vi "lightsource-emission-kill.vi"(1 "NKT Input":T1={"Emission"=FALSE, "Operation Mode"=FALSE, "Power Level"=5.0, "Feedback Level"=0.0, "Short Wavelength (nm)"=560, "Long Wavelength (nm)"=580, "UV Wavelength (nm)"=400} {"UV Wavelength (nm)" min=350 max=480 step=1; "Long Wavelength (nm)" min=400 max=850 step=1; "Short Wavelength (nm)" min=400 max=850 step=1; "Feedback Level" min=0.0 max=90.0 step=0.1 format="%.1f%%"; "Power Level" min=5.0 max=100.0 step=0.1 format="%.1f%%"}, 2 "VISA in":refnum<visa-resource-name>) -> (0 "lightsource init":bool=TRUE)   [LabVIEW 2015]
panel:
  in  "PortParameters":T2={"OpenPort"=FALSE, "ClosePort"=FALSE, "Baudrate"=115200, "Wait"=50, "ReadWrite"=TRUE}
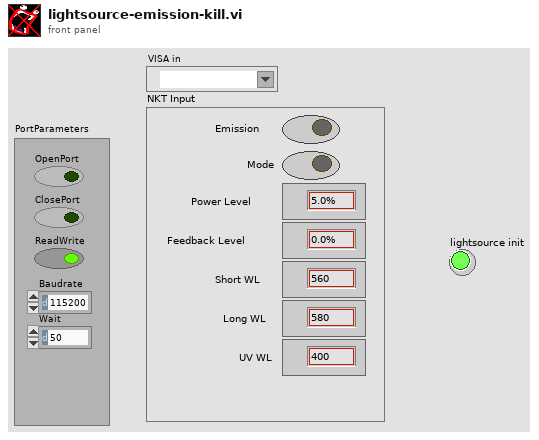
[diagram p1: front panel]
types:
  T1 = cluster{"Emission":bool, "Operation Mode":bool, "Power Level":dbl, "Feedback Level":dbl, "Short Wavelength (nm)":i32, "Long Wavelength (nm)":i32, "UV Wavelength (nm)":i32}
  T2 = cluster{"OpenPort":bool, "ClosePort":bool, "Baudrate":i32, "Wait":u16, "ReadWrite":bool}
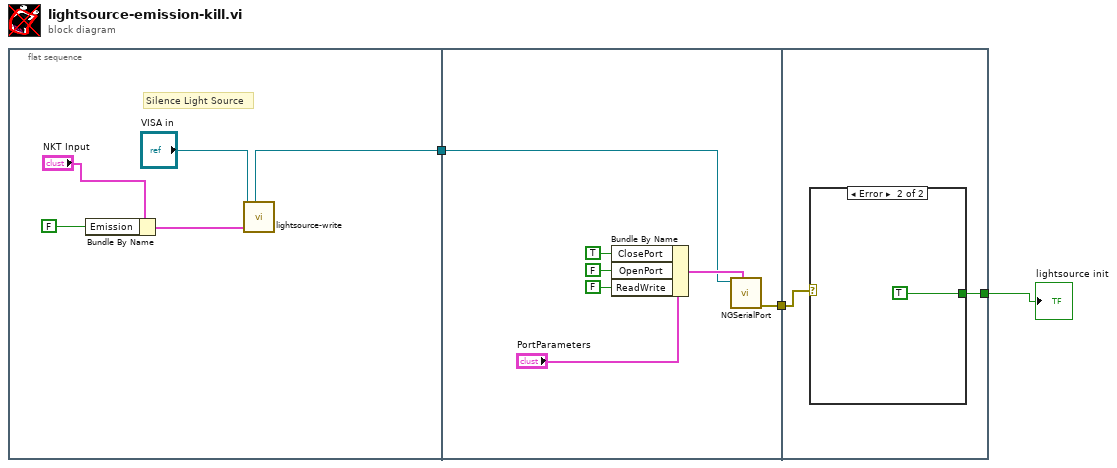
[diagram p0: block diagram]
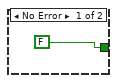
[diagram p2: hidden frame]
diagram:
  n1 = flat-sequence {
    tunnel: [w5] -> w3
    tunnel: w3 -> [w10]
    tunnel: [w9] -> w2
    tunnel: w2 -> [w17]
    tunnel: [w16] -> w1
    frame #0 {
      # "Silence Light Source"
      n2 = Bundle By Name(cluster="NKT Input", "Emission"=FALSE ("Emission On/Off")) -> (w7:T1)
      n3 = call "lightsource-write.vi"("VISA in"="VISA in", "NKT Input"=w7) -> ("VISA out"=w5:refnum<visa-resource-name>)  [unwired: 4 in, 2 out]
    }
    frame #1 {
      n4 = Bundle By Name(cluster="PortParameters", "ClosePort"=TRUE, "OpenPort"=FALSE, "ReadWrite"=FALSE) -> (w11:T2)
      n5 = call "NGSerialPort.vi"("PortParameters"=w11, "VISA in"=w10) -> ("error out"=w9:errorcluster)  [unwired: 7 in, 2 out]
    }
    frame #2 {
      n6 = case shown="Error" w17 {
        tunnel: [FALSE TRUE] -> w16
        frame No Error {
        }
        frame Error {
        }
      }
    }
  }
  "lightsource init" <- w1
